vi "Get_Weight_out_ox_elemetns_at_indexX.vi"(1 "Weights_outX(before being updated)":fxp<+/-,32,8>[][](array[numeric]), 2 "Index":i32) -> (0 "Output_array":fxp<+/-,32,8>[](array[numeric]))   [LabVIEW 2016]
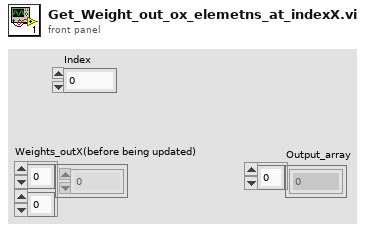
[diagram p1: front panel]
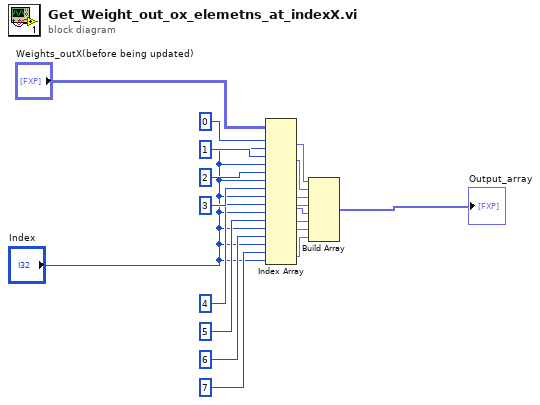
[diagram p0: block diagram]
diagram:
  n1 = Index Array(array="Weights_outX(before being updated)", index (row) #1=0 ("index"), index (col) #1="Index", index (row) #2=1 ("index"), index (col) #2="Index", index (row) #3=2 ("index"), index (col) #3="Index", index (row) #4=3 ("index"), index (col) #4="Index", index (row) #5=4 ("index"), index (col) #5="Index", index (row) #6=5 ("index"), index (col) #6="Index", index (row) #7=6 ("index"), index (col) #7="Index", index (row) #8=7 ("index"), index (col) #8="Index") -> (element #1=w1:fxp<+/-,32,8>, element #2=w9:fxp<+/-,32,8>, element #3=w8:fxp<+/-,32,8>, element #4=w7:fxp<+/-,32,8>, element #5=w6:fxp<+/-,32,8>, element #6=w5:fxp<+/-,32,8>, element #7=w4:fxp<+/-,32,8>, element #8=w3:fxp<+/-,32,8>)
  n2 = Build Array(w1, w9, w8, w7, w6, w5, w4, w3) -> (→"Output_array":fxp<+/-,32,8>[])
